vi "DSO1K Product In XY Mode And Screenshoot.vi"() -> ()   [LabVIEW 2009]
doc: "<B>This VI shows how to use the XY mode, and display the Product Value and screen.</B>"
uses:
  <instrlib>/DSO1K/DSO1K.lvlib
panel:
  in  "Y2 Cursor Position  (-200m)":dbl=-0.2 format="%#_4p"
  in  "Y1 Cursor Position  (200m)":dbl=0.2 format="%#_4p"
  in  "X2 Cursor Position  (200m)":dbl=0.2 format="%#_4p"
  in  "X1 Cursor Position (-200m)":dbl=-0.2 format="%#_4p"
  in  "Timeout (10000ms)":u32=10000
  out "Picture":picture
  out "Product Delta":string
  out "Product Cursor2 Position":string
  out "Product Cursor1 Position":string
  in  "VISA resource name":refnum<visa-resource-name>
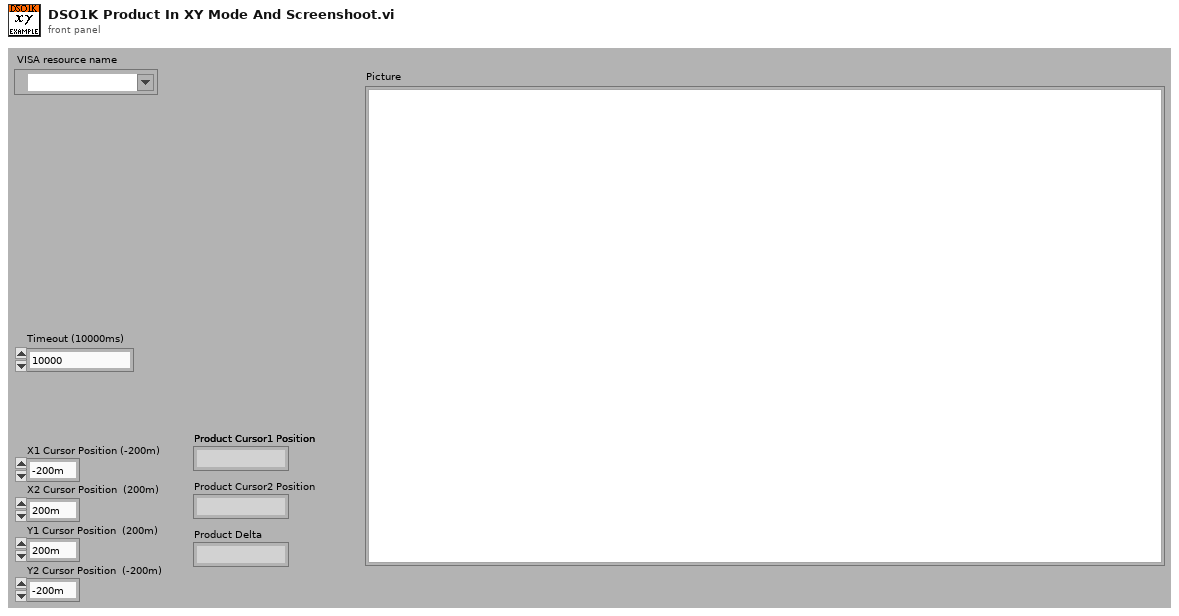
[diagram p1: front panel]
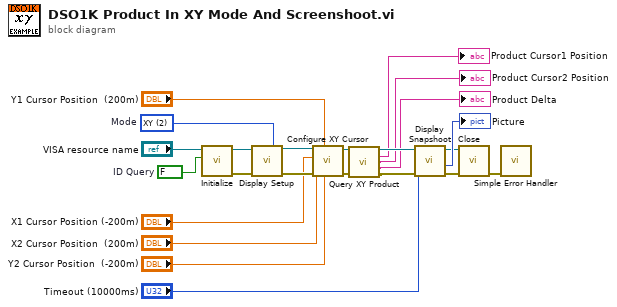
[diagram p0: block diagram]
diagram:
  w12 = u16 2 items=["Main", "Window", "XY"]  # Mode
  w18 = FALSE  # ID Query
  n1 = call <instrlib>:"Initialize.vi"("ID Query (True)"=w18, "VISA resource name"="VISA resource name") -> ("error out"=w21:errorcluster, "VISA resource name out"=w19:refnum<visa-resource-name>)  [unwired: 8 in]
  n2 = call <instrlib>:"Display Setup.vi"("VISA resource name"=w19, "Display Mode (0:Main)"=w12, "error in (no error)"=w21) -> ("VISA resource name out"=w22:refnum<visa-resource-name>, "error out"=w23:errorcluster)  [unwired: 11 in]
  n3 = call <instrlib>:"Configure XY Cursor.vi"("Y2 Cursor Position  (-200m)"="Y2 Cursor Position  (-200m)", "Y1 Cursor Position  (200m)"="Y1 Cursor Position  (200m)", "error in (no error)"=w23, "X2 Cursor Position  (200m)"="X2 Cursor Position  (200m)", "X1 Cursor Position (-200m)"="X1 Cursor Position (-200m)", "VISA resource name"=w22) -> ("error out"=w10:errorcluster, "VISA resource name out"=w11:refnum<visa-resource-name>)  [unwired: 4 in]
  n4 = call <instrlib>:"Query XY Product.vi"("VISA resource name"=w11, "error in (no error)"=w10) -> ("VISA resource name out"=w9:refnum<visa-resource-name>, "Product Cursor1 Position"=→"Product Cursor1 Position":string, "Product Cursor2 Position"=→"Product Cursor2 Position":string, "Product Delta"=→"Product Delta":string, "error out"=w5:errorcluster)  [unwired: 9 in]
  n5 = call <instrlib>:"Display Snapshoot.vi"("error in (no error)"=w5, "Timeout (10000ms)"="Timeout (10000ms)", "VISA resource name"=w9) -> ("error out"=w14:errorcluster, "Picture"=→"Picture":picture, "VISA resource name out"=w15:refnum<visa-resource-name>)  [unwired: 6 in]
  n6 = call <instrlib>:"Close.vi"("error in (no error)"=w14, "VISA resource name"=w15) -> ("error out"=w13:errorcluster)  [unwired: 9 in]
  n7 = call <vilib>:"Simple Error Handler.vi"("error in (no error)"=w13) -> ()  [unwired: 4 in, 5 out]
